vi "loadRoutings.vi"(6 "type":string, 8 "error in (no error)":errorcluster, 9 "device.lvclass":refnum<class "device.lvclass">, 10 "channel_configXML":refnum<class "NativeXML.lvclass">, 11 "deviceDataBase in":refnum<class "deviceDataBase.lvclass">) -> (0 "error out":errorcluster, 1 "device.lvclass out":refnum<class "device.lvclass">, 2 "channel_configXML":refnum<class "NativeXML.lvclass">, 3 "deviceDataBase out":refnum<class "deviceDataBase.lvclass">)   [LabVIEW 2011, in "Tools.lvlib" / "DatabaseHelpers.lvlib" / "deviceDataBase.lvclass"]
uses:
  deviceDataBase.lvclass
  NativeXML/NativeXML.lvclass
  Database Objects/device/device.lvclass
  Database Objects/device/DigitalDevice/DigitalDevice.lvclass
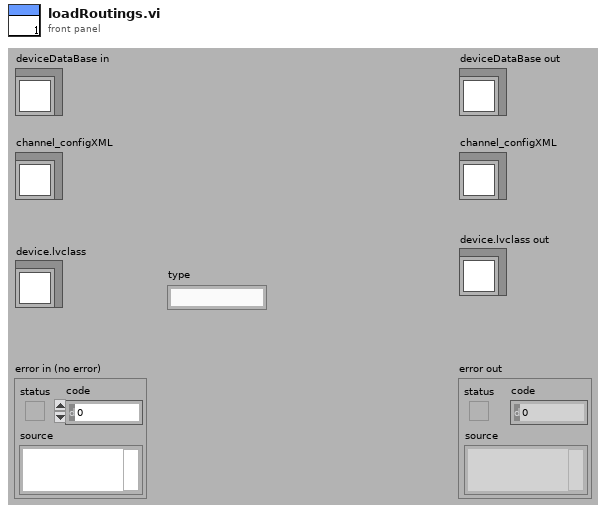
[diagram p1: front panel]
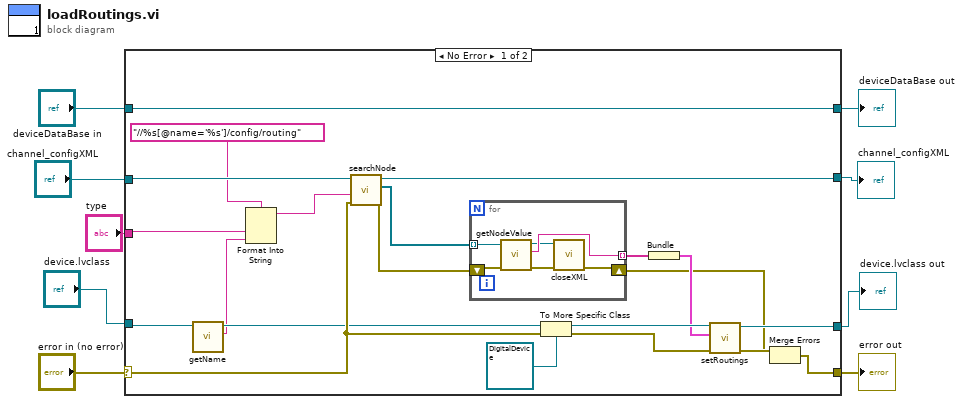
[diagram p0: block diagram]
diagram:
  n1 = case shown="No Error" "error in (no error)" {
    selector: "error in (no error)" -> [w18 w38]
    tunnel: [w21 w38] -> w8
    tunnel: [w30 w37] -> w6
    tunnel: "deviceDataBase in" -> [w30 w37]
    tunnel: "channel_configXML" -> [w19 _]
    tunnel: "device.lvclass" -> [w16 _]
    tunnel: [w20 _] -> w3
    tunnel: [w24 _] -> w2
    tunnel: "type" -> [w14 _]
    frame No Error {
      n2 = call "getName.vi"("device.lvclass in"=w16) -> ("name"=w13:string, "device.lvclass out"=w15:refnum<class "device.lvclass">)  [unwired: 8 in, 1 out]
      n3 = Format Into String(format string="//%s[@name='%s']/config/routing", w14, w13) -> (resulting string=w10:string)  [unwired: 2 in, 1 out]
      n4 = call "searchNode.vi"("error in (no error)"=w18, "searchXPath"=w10, "NativeXML in"=w19) -> ("error out"=w17:errorcluster, "nodeArray"=w11:refnum<class "NativeXML.lvclass">[], "NativeXML out"=w20:refnum<class "NativeXML.lvclass">)  [unwired: 6 in]
      n5 = for {
        tunnel: w11 -> [w35] mode=indexing
        shift-right: [w31] -> w22
        shift-left: w17 -> [w36]
        tunnel: [w34] -> w26 mode=indexing
        n6 = call "getNodeValue.vi"("error in (no error)"=w36, "NativeXML in"=w35) -> ("error out"=w32:errorcluster, "Value"=w34:string, "NativeXML out"=w33:refnum<class "NativeXML.lvclass">)  [unwired: 7 in]
        n7 = call "closeXML.vi"("error in (no error)"=w32, "NativeXML in"=w33) -> ("error out"=w31:errorcluster)  [unwired: 9 in]
      }
      n8 = To More Specific Class(target class=refnum<class "DigitalDevice.lvclass"> refnum ("DigitalDevice.lvclass in"), reference=w15, error in=w18) -> (specific class reference=w28:refnum<class "DigitalDevice.lvclass">, error out=w27:errorcluster)
      n9 = Bundle(w26) -> (w25:cluster{string[]})  [unwired: 1 in]
      n10 = call "setRoutings.vi"("error in (no error)"=w27, "Routings"=w25, "DigitalDevice.lvclass in"=w28) -> ("error out"=w23:errorcluster, "DigitalDevice.lvclass out"=w24:refnum<class "DigitalDevice.lvclass">)  [unwired: 7 in]
      n11 = Merge Errors(w22, w23) -> (w21:errorcluster)
    }
    frame Error {
    }
  }
  "error out" <- w8
  "deviceDataBase out" <- w6
  "device.lvclass out" <- w2
  "channel_configXML" <- w3
